vi "RealTimeNeph.vi"(8 "error in (no error)":errorcluster) -> (0 "error out":errorcluster)   [LabVIEW 2013]
doc: "Use this template to build a VI to use as a subVI."
uses:
  <vilib>/Instr/_visa.llb/VISA Configure Serial Port (Instr).vi
  <vilib>/Utility/file.llb/Write To Spreadsheet File (string).vi
  <vilib>/ptbypt/NI_PtbyPt.lvlib
panel:
  out "Total Scattering (Red (632nm), Green (532nm), Blue (450nm))":T1(graph)={"Numeric"=11.768620561478, "Numeric"=10.3616270811, "Numeric"=32.318224076812}
  out "Temperature":dbl(graph)=24.22
  out "Pressure":dbl(graph)=101.15
  out "Humidity":dbl(graph)=48.6
  in  "Include Averages and Std":bool=TRUE
  in  "sample length":i32=38
  in  "Nephelometer Com Port":refnum<visa-resource-name>="COM16"
  in  "Save To File":bool=TRUE
  in  "File Path Control":path=path "T:/LabBox/Software/Airphoton Nephelometer/TestMean.csv"
  in  "Array":dbl[](array[numeric])
  in  "stop":bool
  out "read buffer":string="IN1024,9/17/15 10:52:54,3093186,10310875,2353742,4299422,4381491,6981848,1595346,20761660,1351020,7590174,2065561,14187844,24.22,101.15,48.6,874857,984521,1006387,4.775941096085,5.786920205497,5.869425532089,11.768620561478,10.361627081100,32.318224076812,0\u0000"
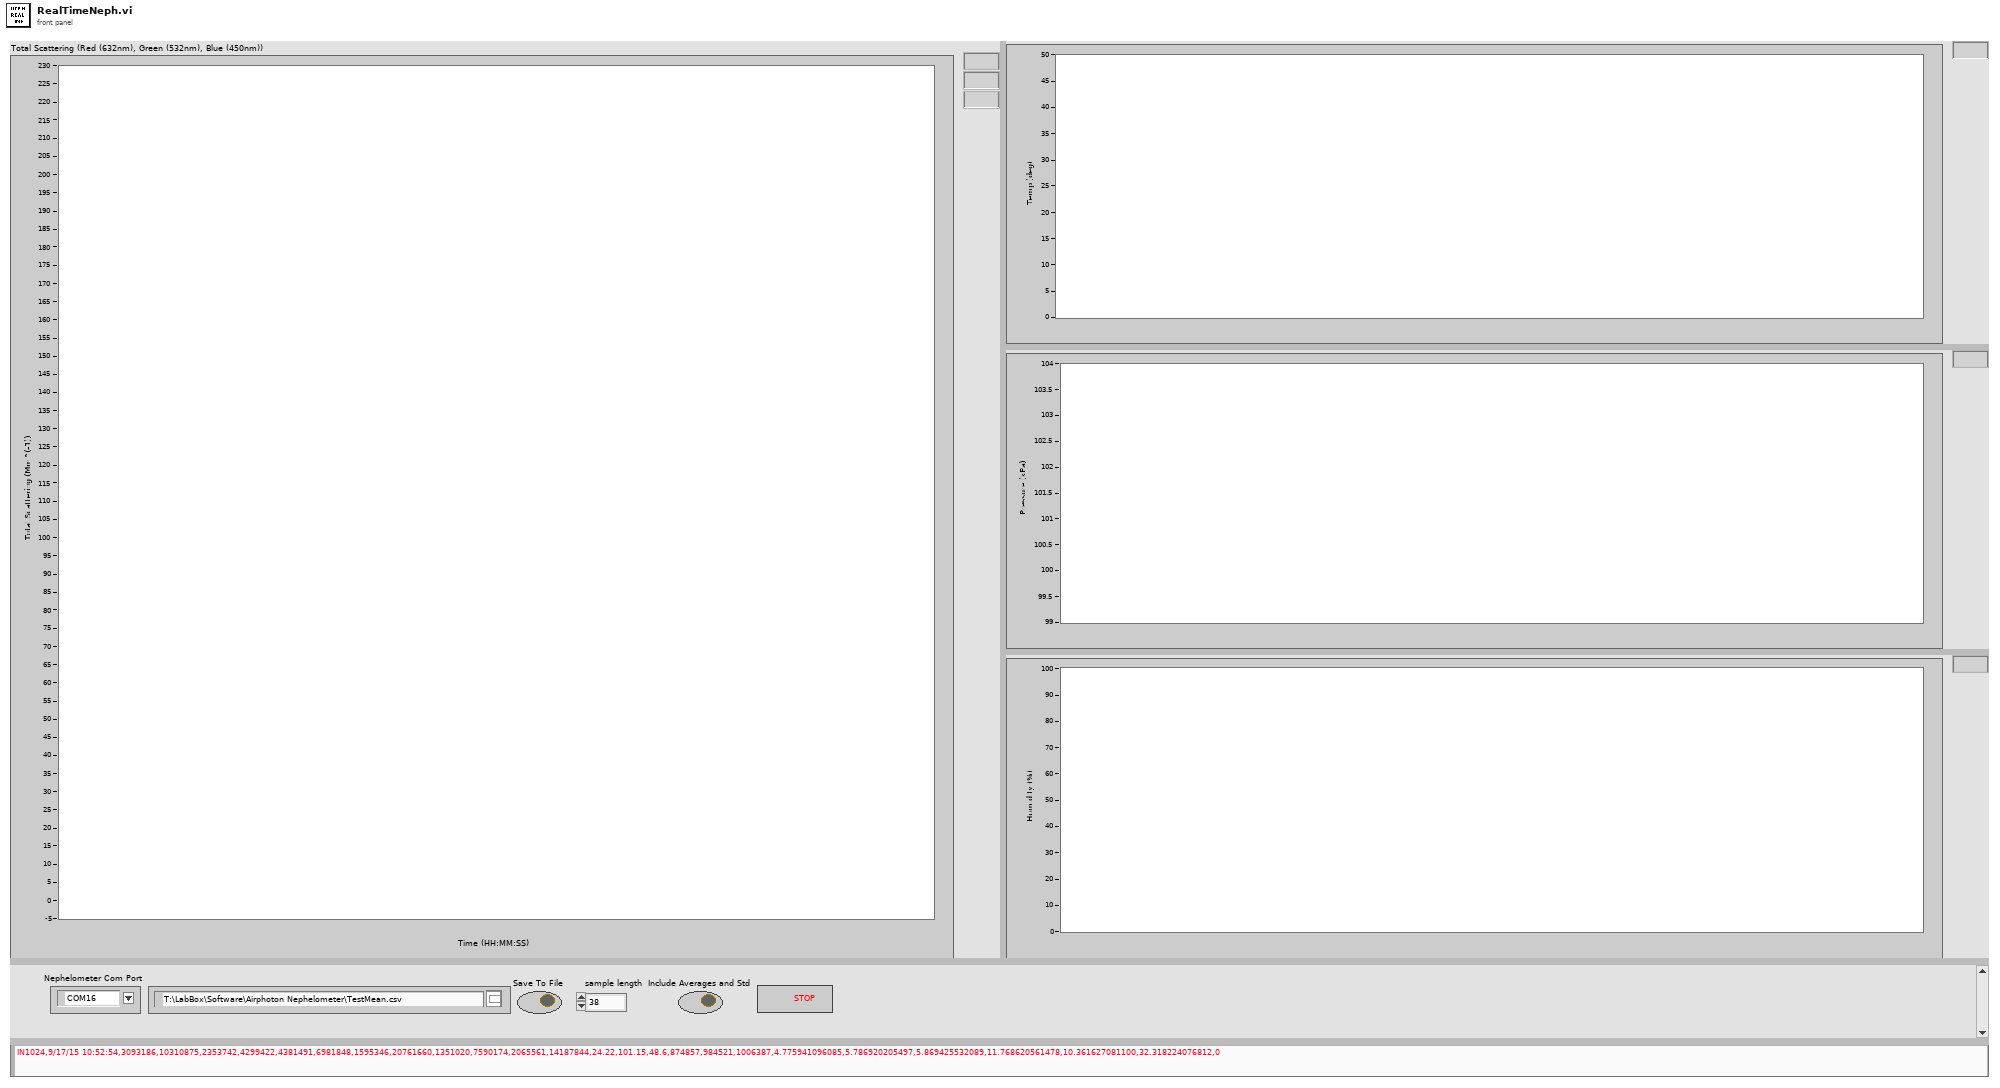
[diagram p1: front panel]
types:
  T1 = cluster{"Numeric":dbl, "Numeric":dbl, "Numeric":dbl}
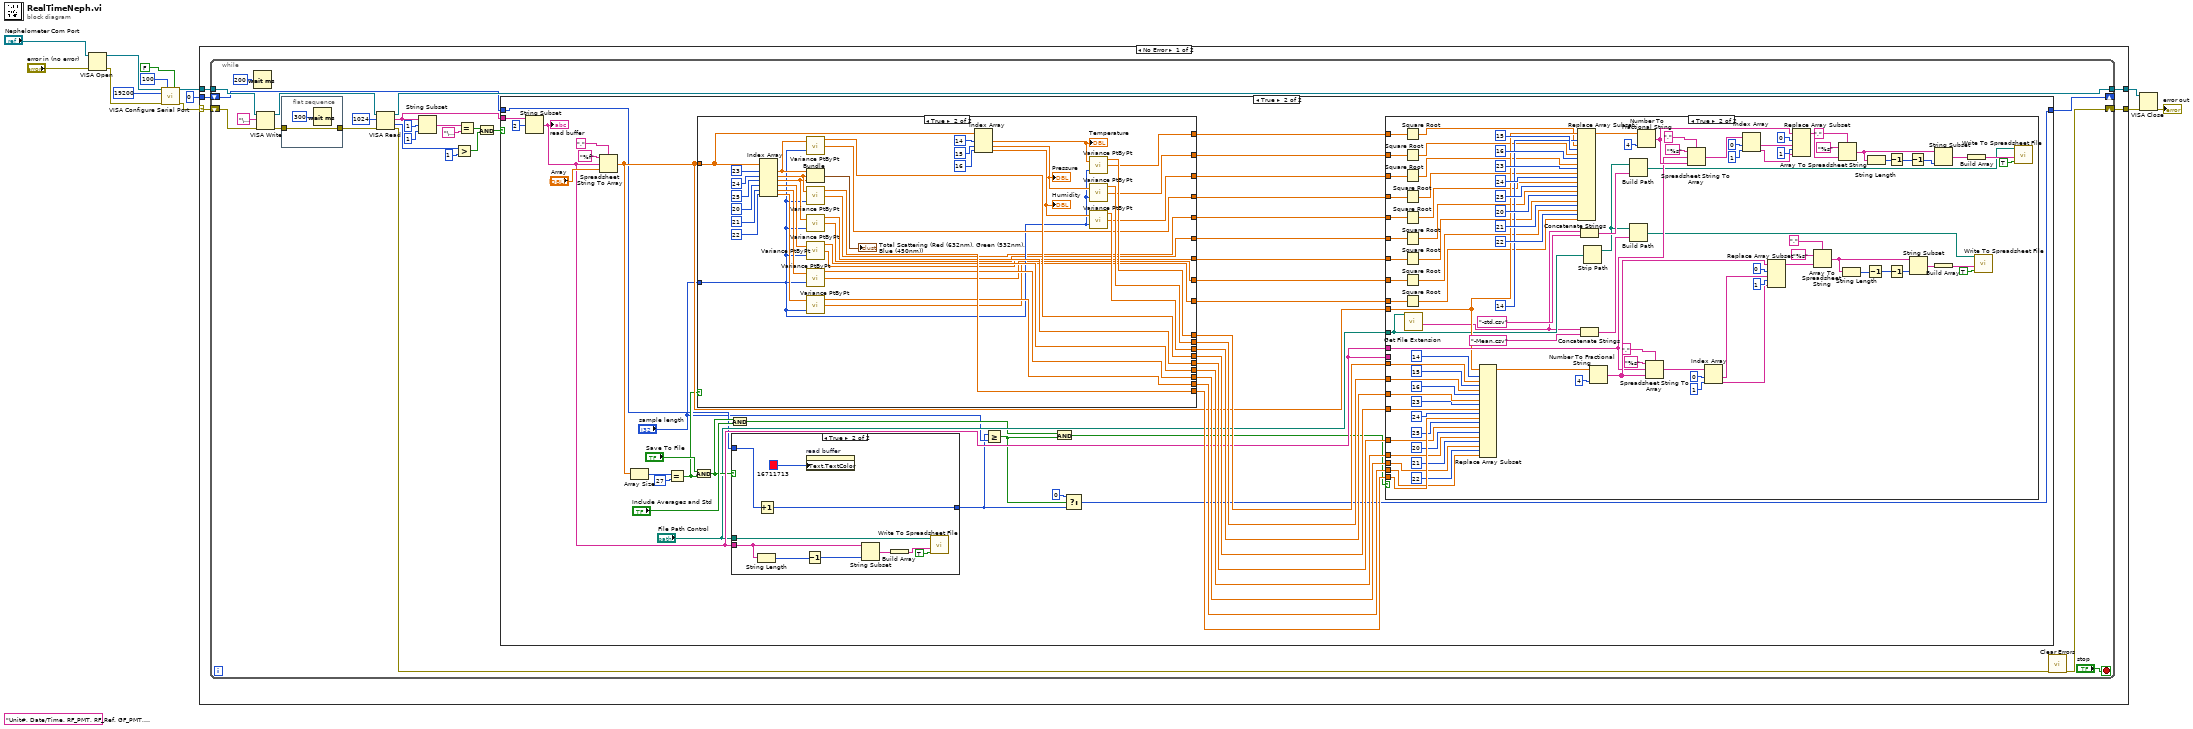
[diagram p0: block diagram]
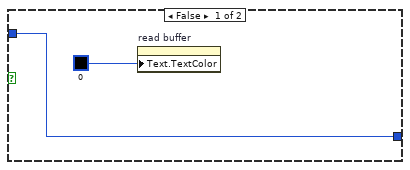
[diagram p4: hidden frame]
diagram:
  (unwired) "Unit#, Date/Time, RF_PMT, RF_Ref, GF_PMT, GF_REF, BF_PMT, BF_REF, RB_PMT, RB_REF, GB_PMT, GB_REF, BB_PMT, BB_REF,Temp ,Pressure, RH%,  PMT DARK, Forw Dark Ref, Back Dark Ref, Back scatt Red, Back scatt Green, Back scatt Blue , Total scatt Red, Total scatt Green, Total scatt Blue, Fan RPM" ("write buffer")
  n1 = VISA Open(error in (no error)="error in (no error)", VISA resource name="Nephelometer Com Port") -> (VISA resource name=w7:refnum<visa-resource-name>, error out=w6:errorcluster)  [unwired: 3 in]
  n2 = call-poly "VISA Configure Serial Port"("VISA resource name"=w7, "timeout (10sec)"=u32 100, "Enable Termination\nChar (T)"=FALSE ("Enable Termination\nChar (T)"), "baud rate (9600)"=u32 19200, "error in (no error)"=w6) -> ("VISA resource name out"=w9:refnum<visa-resource-name>, "error out"=w10:errorcluster)  [unwired: 9 in]
  n3 = case shown="No Error" w10 {
    selector: w10 -> [w17 w238]
    tunnel: [w16 w238] -> w12
    tunnel: [w15 w237] -> w13
    tunnel: w9 -> [w18 w237]
    tunnel: 0 -> [w14 _]
    frame No Error {
      n4 = while {
        tunnel: w18 -> [w42]
        shift-right: [w33] -> w16
        shift-left: w17 -> [w41]
        tunnel: [w35] -> w15
        shift-right: [w21] -> _
        shift-left: w14 -> [w22]
        stop <- "stop" stop-if-true
        n5 = Wait (ms)(milliseconds to wait=u32 200) -> ()  [unwired: 1 out]
        n6 = VISA Write(VISA resource name=w42, write buffer="\u0005", error in (no error)=w41) -> (VISA resource name out=w40:refnum<visa-resource-name>, error out=w20:errorcluster)  [unwired: 1 out]
        n7 = flat-sequence {
          tunnel: w20 -> [w43]
          tunnel: [w43] -> w19
          frame #0 {
            n8 = Wait (ms)(milliseconds to wait=u32 300) -> ()  [unwired: 1 out]
          }
        }
        n9 = VISA Read(VISA resource name=w40, byte count=u32 1024, error in (no error)=w19) -> (VISA resource name out=w35:refnum<visa-resource-name>, read buffer=w30:string, return count=w32:u32, error out=w34:errorcluster)
        n10 = String Subset(string=w30, offset (0)=1, length (rest)=1 ("length (rest)")) -> (substring=w28:string)
        n11 = Greater?(x=w32, y=u32 1) -> (0:w25:bool)
        n12 = Equal?(x=w28, y="\u0006" ("write buffer")) -> (x = y?=w26:bool)
        n13 = And(x=w26, y=w25) -> (x .and. y?=w24:bool)
        n14 = case shown="True" w24 {
          tunnel: w30 -> [_ w85]
          tunnel: w22 -> [w45 w53]
          tunnel: [w45 w47] -> w21
          frame False {
          }
          frame True {
            n15 = String Subset(string=w85, offset (0)=2) -> (substring=w59:string)  [unwired: 1 in]
            "read buffer" <- w59
            n16 = Spreadsheet String To Array(delimiter (Tab)=",", format string="%f", spreadsheet string=w59, array type (2D Dbl)="Array") -> (array=w62:dbl[])
            n17 = Array Size(array=w62) -> (size(s)=w61:i32)
            n18 = Equal?(x=w61, y=27) -> (x = y?=w54:bool)
            n19 = And(x="Save To File", y=w54) -> (x .and. y?=w57:bool)
            n20 = case shown="True" w54 {
              tunnel: [_ w105] -> w80
              tunnel: [_ w104] -> w79
              tunnel: [_ w103] -> w78
              tunnel: [_ w102] -> w77
              tunnel: [_ w101] -> w76
              tunnel: [_ w100] -> w75
              tunnel: [_ w99] -> w74
              tunnel: [_ w98] -> w73
              tunnel: [_ w97] -> w72
              tunnel: [_ w96] -> w71
              tunnel: [_ w95] -> w70
              tunnel: [_ w94] -> w69
              tunnel: [_ w93] -> w68
              tunnel: [_ w90] -> w67
              tunnel: [_ w89] -> w66
              tunnel: [_ w88] -> w65
              tunnel: [_ w87] -> w64
              tunnel: [_ w86] -> w63
              tunnel: w62 -> [_ w92]
              tunnel: "sample length" -> [_ w91]
              frame False {
              }
              frame True {
                n21 = Index Array(array=w92, index #1=23 ("index"), index #2=24 ("index"), index #3=25 ("index"), index #4=20 ("index"), index #5=21 ("index"), index #6=22 ("index")) -> (element #1=w108:dbl, element #2=w107:dbl, element #3=w106:dbl, element #4=w111:dbl, element #5=w110:dbl, element #6=w109:dbl)
                n22 = call <vilib>:"Variance PtByPt.vi"("x"=w108, "sample length"=w91) -> ("mean"=w102:dbl, "variance"=w93:dbl)  [unwired: 1 in, 1 out]
                n23 = Bundle("Numeric"=w108, "Numeric"=w107, "Numeric"=w106) -> (→"Total Scattering (Red (632nm), Green (532nm), Blue (450nm))":T1)  [unwired: 1 in]
                n24 = call <vilib>:"Variance PtByPt.vi"("x"=w107, "sample length"=w91) -> ("mean"=w101:dbl, "variance"=w90:dbl)  [unwired: 1 in, 1 out]
                n25 = call <vilib>:"Variance PtByPt.vi"("x"=w106, "sample length"=w91) -> ("mean"=w100:dbl, "variance"=w89:dbl)  [unwired: 1 in, 1 out]
                n26 = call <vilib>:"Variance PtByPt.vi"("x"=w111, "sample length"=w91) -> ("mean"=w99:dbl, "variance"=w88:dbl)  [unwired: 1 in, 1 out]
                n27 = call <vilib>:"Variance PtByPt.vi"("x"=w110, "sample length"=w91) -> ("mean"=w98:dbl, "variance"=w87:dbl)  [unwired: 1 in, 1 out]
                n28 = call <vilib>:"Variance PtByPt.vi"("x"=w109, "sample length"=w91) -> ("mean"=w97:dbl, "variance"=w86:dbl)  [unwired: 1 in, 1 out]
                n29 = Index Array(array=w92, index #1=14 ("index"), index #2=15 ("index"), index #3=16 ("index")) -> (element #1=w117:dbl, element #2=w116:dbl, element #3=w115:dbl)
                "Temperature" <- w117
                "Pressure" <- w116
                "Humidity" <- w115
                n30 = call <vilib>:"Variance PtByPt.vi"("x"=w117, "sample length"=w91) -> ("mean"=w105:dbl, "variance"=w96:dbl)  [unwired: 1 in, 1 out]
                n31 = call <vilib>:"Variance PtByPt.vi"("x"=w116, "sample length"=w91) -> ("mean"=w104:dbl, "variance"=w95:dbl)  [unwired: 1 in, 1 out]
                n32 = call <vilib>:"Variance PtByPt.vi"("x"=w115, "sample length"=w91) -> ("mean"=w103:dbl, "variance"=w94:dbl)  [unwired: 1 in, 1 out]
              }
            }
            n33 = And(x=w57, y="Include Averages and Std") -> (x .and. y?=w52:bool)
            n34 = case shown="True" w57 {
              tunnel: w59 -> [_ w131]
              tunnel: "File Path Control" -> [_ w130]
              tunnel: w53 -> [w126 w129]
              tunnel: [w126 w128] -> w46
              frame False {
                n35 = property on="read buffer" class="Str"("Text.TextColor"=u32 0) -> ()  [unwired: 2 in, 2 out]
              }
              frame True {
                n36 = String Length(string=w131) -> (length=w135:i32)
                n37 = Increment(x=w129) -> (x+1=w128:i32)
                n38 = Decrement(x=w135) -> (x-1=w134:i32)
                n39 = property on="read buffer" class="Str"("Text.TextColor"=u32 16711713) -> ()  [unwired: 2 in, 2 out]
                n40 = String Subset(string=w131, length (rest)=w134) -> (substring=w133:string)  [unwired: 1 in]
                n41 = Build Array(w133) -> (w132:string[])
                n42 = call-poly <vilib>:"Write To Spreadsheet File.vi"("append to file? (new file:F)"=TRUE, "1D data"=w132, "file path (dialog if empty)"=w130) -> ()  [unwired: 5 in, 1 out]
              }
            }
            n43 = Greater Or Equal?(x=w46, y="sample length") -> (x >= y?=w49:bool)
            n44 = And(x=w52, y=w49) -> (x .and. y?=w51:bool)
            n45 = Select(t=0, s=w49, f=w46) -> (s? t:f=w47:i32)
            n46 = case shown="True" w51 {
              tunnel: w59 -> [_ _]
              tunnel: w80 -> [_ w236]
              tunnel: w79 -> [_ w235]
              tunnel: w78 -> [_ w234]
              tunnel: w77 -> [_ w233]
              tunnel: w76 -> [_ w232]
              tunnel: w75 -> [_ w231]
              tunnel: w74 -> [_ w230]
              tunnel: w73 -> [_ w229]
              tunnel: w72 -> [_ w228]
              tunnel: w62 -> [_ w178]
              tunnel: w59 -> [_ w179]
              tunnel: w71 -> [_ w168]
              tunnel: w70 -> [_ w167]
              tunnel: w69 -> [_ w166]
              tunnel: w68 -> [_ w165]
              tunnel: w67 -> [_ w164]
              tunnel: w66 -> [_ w163]
              tunnel: w65 -> [_ w162]
              tunnel: w64 -> [_ w161]
              tunnel: w63 -> [_ w160]
              tunnel: "File Path Control" -> [_ w159]
              frame False {
              }
              frame True {
                n47 = Square Root(x=w168) -> (sqrt(x)=w177:dbl)
                n48 = Square Root(x=w167) -> (sqrt(x)=w176:dbl)
                n49 = Square Root(x=w166) -> (sqrt(x)=w175:dbl)
                n50 = Square Root(x=w165) -> (sqrt(x)=w174:dbl)
                n51 = Square Root(x=w164) -> (sqrt(x)=w173:dbl)
                n52 = Square Root(x=w163) -> (sqrt(x)=w172:dbl)
                n53 = Square Root(x=w162) -> (sqrt(x)=w171:dbl)
                n54 = Square Root(x=w161) -> (sqrt(x)=w170:dbl)
                n55 = Square Root(x=w160) -> (sqrt(x)=w169:dbl)
                n56 = call <vilib>:"Get File Extension.vi"("file"=w159) -> ("filename without extension"=w155:string)  [unwired: 7 in, 3 out]
                n57 = Replace Array Subset(array=w178, new element #1=w236, index #1=14 ("index"), new element #2=w235, index #2=15 ("index"), new element #3=w234, index #3=16 ("index"), new element #4=w233, index #4=23 ("index"), new element #5=w232, index #5=24 ("index"), new element #6=w231, index #6=25 ("index"), new element #7=w230, index #7=20 ("index"), new element #8=w229, index #8=21 ("index"), new element #9=w228, index #9=22 ("index")) -> (w218:dbl[])
                n58 = Replace Array Subset(array=w178, new element #1=w177, index #1=14 ("index"), new element #2=w176, index #2=15 ("index"), new element #3=w175, index #3=16 ("index"), new element #4=w174, index #4=23 ("index"), new element #5=w173, index #5=24 ("index"), new element #6=w172, index #6=25 ("index"), new element #7=w171, index #7=20 ("index"), new element #8=w170, index #8=21 ("index"), new element #9=w169, index #9=22 ("index")) -> (w189:dbl[])
                n59 = Concatenate Strings(w155, "-std.csv" ("string")) -> (w154:string)
                n60 = Concatenate Strings(w155, "-Mean.csv" ("string")) -> (w157:string)
                n61 = Strip Path(path=w159) -> (stripped path=w153:path)  [unwired: 1 out]
                n62 = Number To Fractional String(number=w218, precision (6)=i16 4) -> (F-format string=w210:string[])  [unwired: 2 in]
                n63 = Build Path(base path=w153, name or relative path=w154) -> (appended path=w148:path)
                n64 = Build Path(base path=w153, name or relative path=w157) -> (appended path=w147:path)
                n65 = Number To Fractional String(number=w189, precision (6)=i16 4) -> (F-format string=w197:string[])  [unwired: 2 in]
                n66 = Spreadsheet String To Array(delimiter (Tab)=",", format string="%s", spreadsheet string=w179, array type (2D Dbl)=w210) -> (array=w209:string[])
                n67 = Spreadsheet String To Array(delimiter (Tab)=",", format string="%s", spreadsheet string=w179, array type (2D Dbl)=w197) -> (array=w198:string[])
                n68 = Index Array(array=w209, index #1=0 ("index"), index #2=1 ("index")) -> (element #1=w206:string, element #2=w205:string)
                n69 = Index Array(array=w198, index #1=0 ("index"), index #2=1 ("index")) -> (element #1=w201:string, element #2=w202:string)
                n70 = Replace Array Subset(array=w210, new element #1=w206, index #1=0 ("index"), new element #2=w205, index #2=1 ("index")) -> (w204:string[])
                n71 = Replace Array Subset(array=w197, new element #1=w201, index #1=0 ("index"), new element #2=w202, index #2=1 ("index")) -> (w203:string[])
                n72 = Array To Spreadsheet String(delimiter (Tab)=",", array=w204, 3:"%s" ("format string")) -> (spreadsheet string=w145:string)
                n73 = Array To Spreadsheet String(delimiter (Tab)=",", array=w203, 3:"%s" ("format string")) -> (spreadsheet string=w142:string)
                n74 = String Length(string=w145) -> (length=w146:i32)
                n75 = Decrement(x=w146) -> (x-1=w140:i32)
                n76 = String Length(string=w142) -> (length=w143:i32)
                n77 = Decrement(x=w143) -> (x-1=w138:i32)
                n78 = Decrement(x=w140) -> (x-1=w139:i32)
                n79 = Decrement(x=w138) -> (x-1=w137:i32)
                n80 = String Subset(string=w145, length (rest)=w139) -> (substring=w144:string)  [unwired: 1 in]
                n81 = String Subset(string=w142, length (rest)=w137) -> (substring=w141:string)  [unwired: 1 in]
                n82 = Build Array(w144) -> (w149:string[])
                n83 = Build Array(w141) -> (w152:string[])
                n84 = call-poly <vilib>:"Write To Spreadsheet File.vi"("append to file? (new file:F)"=TRUE, "1D data"=w149, "file path (dialog if empty)"=w147) -> ()  [unwired: 5 in, 1 out]
                n85 = call-poly <vilib>:"Write To Spreadsheet File.vi"("append to file? (new file:F)"=TRUE, "1D data"=w152, "file path (dialog if empty)"=w148) -> ()  [unwired: 5 in, 1 out]
              }
            }
          }
        }
        n86 = call <vilib>:"Clear Errors.vi"("error in (no error)"=w34) -> ("error out"=w33:errorcluster)  [unwired: 6 in]
      }
    }
    frame Error {
    }
  }
  n87 = VISA Close(VISA resource name=w13, error in (no error)=w12) -> (error out=→"error out":errorcluster)
